vi "get_active_application_list.vi"(8 "error in":errorcluster, 11 "path in":path) -> (0 "error out":errorcluster, 1 "ATSMasterAppNames":string, 2 "return":i32, 3 "path out":path)   [LabVIEW 2014]
doc: "Function introduction: Obtain CAN database information\nCall location\nInput parameter ADatabaseId: Database ID AType: Type\nAIndes: Database Index\nASUbIndex: CAN Index\nAvalue: Real Value\nReturn value==0: Successful execution\nOther values: Query error code"
uses:
  <vilib>/Utility/importsl/GetValueByPointer/GetValueByPointer.xnode
  <vilib>/Utility/importsl/GetValueByPointer/datatype.ctl
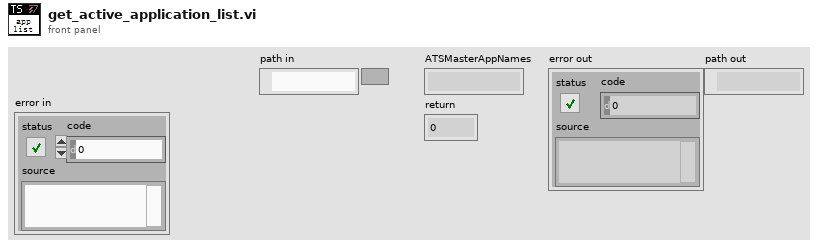
[diagram p1: front panel]
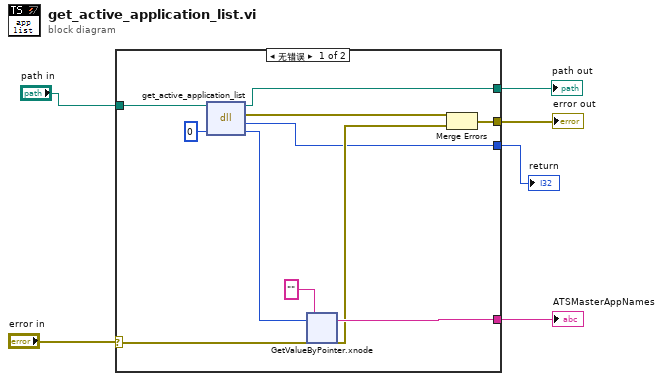
[diagram p0: block diagram]
diagram:
  n1 = case shown="无错误" "error in" {
    selector: "error in" -> [w15 w31]
    tunnel: [w12 _] -> w6
    tunnel: [w13 w31] -> w4
    tunnel: "path in" -> [w10 w30]
    tunnel: [w9 w30] -> w2
    tunnel: [w8 _] -> w1
    frame No Error {
      n2 = dll-call lib="D:/Program Files (x86)/TOSUN/TSMaster/bin64/TSMaster.dll" fn="get_active_application_list"(path in=w10, "ATSMasterAppNames"=u64 0) -> (path out=w9:path, error out=w14:errorcluster, "ACode"=w8:i32, "ATSMasterAppNames"=w17:u64)  [unwired: 2 in]
      n3 = xnode "GetValueByPointer.xnode"("Pointer"=w17, "InputType"="", "ErrorIn"=w15) -> ("Output"=w12:string, "ErrorOut"=w11:errorcluster)  [unwired: 1 in]
      n4 = Merge Errors(w14, w11) -> (w13:errorcluster)
    }
    frame Error {
    }
  }
  "error out" <- w4
  "ATSMasterAppNames" <- w6
  "path out" <- w2
  "return" <- w1
